vi "XIPIN_Video_Scaler_8_1.vi"   [LabVIEW 2017]
doc: "Discontinued. Please select the Video Processing Subsystem.\n------------------------------------\n<b>Need License</b> : Yes\n<b>Interface</b> : AXI4 AXI4-Stream"
uses:
  <vilib>/rvi/XilinxIP/XIPIN_XNode/niFpgaXIPIN.xnode
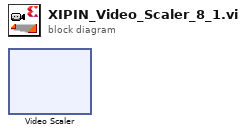
[diagram p0: block diagram]
diagram:
  n1 = xnode ("Video Scaler")() -> ()
